vi "Rotate Array.vi"(1 "Rotation Orientation":bool, 2 "Rotation":enum8{"90", "180", "270"}(ring), 3 "Array":u8[][](array[numeric])=[[0, 1, 2, 12], [3, 4, 5, 12], [6, 7, 8, 12], [9, 10, 11, 12]]) -> (0 "Rotated 2D Array":u8[][](array[numeric]))   [LabVIEW 2014]
doc: "This VI rotates a 2D array in either clockwise or clockwise by a multiple of 90 degrees."
panel:
  # "This VI rotates a 2D array either clockwise or counterclockwise by\n90, 180, or 270 degrees."
  # "Clockwise\n\nCounterclockwise"
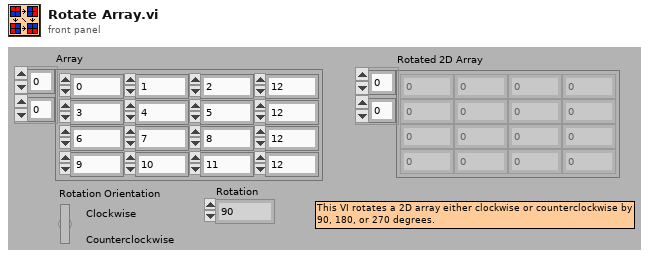
[diagram p1: front panel]
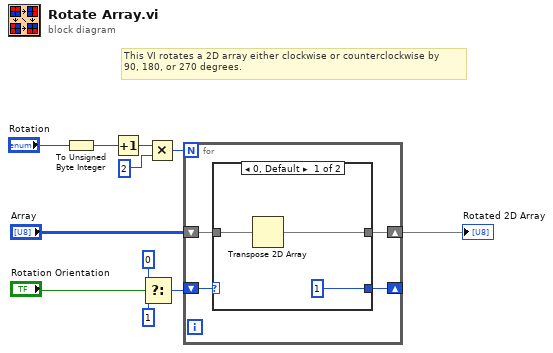
[diagram p0: block diagram]
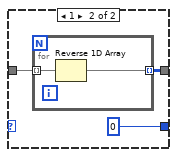
[diagram p2: hidden frame]
diagram:
  # "This VI rotates a 2D array either clockwise or counterclockwise by\n90, 180, or 270 degrees."
  n1 = To Unsigned Byte Integer(number="Rotation") -> (unsigned 8bit integer=w1:u8)
  n2 = Increment(x=w1) -> (x+1=w3:u8)
  n3 = Select(t=u8 0, s="Rotation Orientation", f=u8 1) -> (s? t:f=w5:u8)
  n4 = Multiply(x=w3, y=u8 2) -> (x*y=w4:u8)
  n5 = for {
    N: w4 -> [_]
    shift-right: [w14] -> w10
    shift-left: "Array" -> [w15]
    shift-right: [w12] -> _
    shift-left: w5 -> [w13]
    n6 = case shown="0, Default" w13 {
      tunnel: w15 -> [w17 w21]
      tunnel: [w18 w20] -> w14
      tunnel: [u8 1 u8 0] -> w12
      frame 0, Default {
        n7 = Transpose 2D Array(2D array=w17) -> (transposed array=w18:u8[][])
      }
      frame 1 {
        n8 = for {
          tunnel: w21 -> [w23] mode=indexing
          tunnel: [w22] -> w20 mode=indexing
          n9 = Reverse 1D Array(array=w23) -> (reversed array=w22:u8[])
        }
      }
    }
  }
  "Rotated 2D Array" <- w10
